vi "Pre Launch Init.vi"(11 "CameraTesting in":refnum<class "CameraTesting.lvclass">) -> (0 "error out":errorcluster, 3 "CameraTesting out":refnum<class "CameraTesting.lvclass">)   [LabVIEW 2020, in "CameraTesting.lvlib" / "CameraTesting.lvclass"]
doc: "(<B>Filename</B>: Actor Framework.lvlib:Actor.lvclass:Pre Launch Init.vi)\n\nDefines behavior that occurs after the Launch Nested Actor method is invoked but before the actor's Actor Core method begins running.\n\nBy default, this method does nothing. A descendant class may override it to define behavior."
uses:
  CameraTesting.lvclass
  CameraTesting.lvclass/CameraTesting.ctl
  <vilib>/ActorFramework/Actor/Actor.lvclass
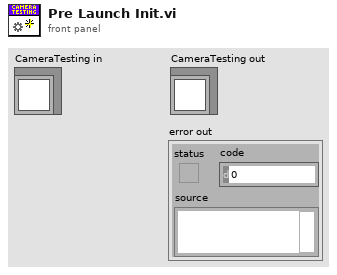
[diagram p1: front panel]
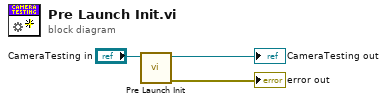
[diagram p0: block diagram]
diagram:
  n1 = call-parent "Pre Launch Init.vi"("Actor in"="CameraTesting in") -> ("error out"=→"error out":errorcluster, "Actor out"=→"CameraTesting out":refnum<class "CameraTesting.lvclass">)  [unwired: 9 in]
